vi "string to 2 digit hex.vi"(8 "error in":errorcluster, 11 "string in":string) -> (0 "error out":errorcluster, 1 "remaining string":string, 2 "output 1":T1 format="0x%02x", 3 "Numeric":i32)   [LabVIEW 2016]
uses:
  2 digit hex indicator.ctl
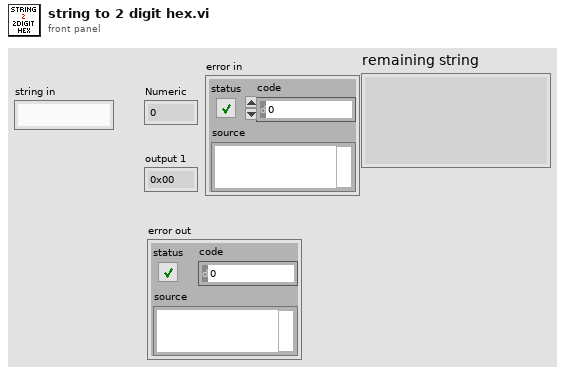
[diagram p1: front panel]
types:
  T1 = typedef "2 digit hex indicator.ctl" = i32
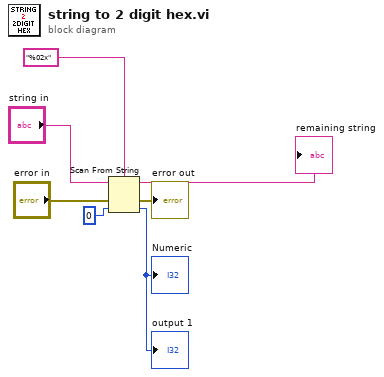
[diagram p0: block diagram]
diagram:
  n1 = Scan From String(format string="%02x", input string="string in", error in="error in", default 1=0) -> (remaining string=→"remaining string":string, error out=→"error out":errorcluster, output 1=→"output 1" →"Numeric":i32)  [unwired: 1 in, 1 out]
